vi "EOD Read TEST.vi"(8 "error in (no error)":errorcluster, 11 "Byte Stream File in":refnum<file>) -> (0 "error out":errorcluster, 1 "EODDataOut":T1(array[cluster]), 2 "Iteration Number":i32, 3 "Byte Stream File out":refnum<file>)   [LabVIEW 2014]
panel:
  out "Wave Offset":i32[](array[numeric])
  # "EOD File Reader VI"
  # "Inputs"
  # "Outputs"
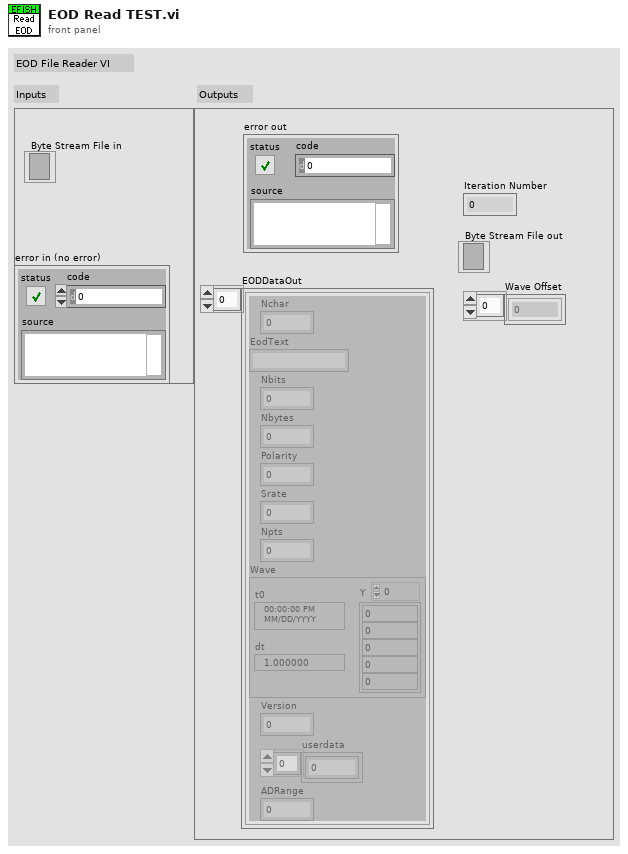
[diagram p1: front panel]
types:
  T1 = cluster{"Nchar":i32, "EodText":string, "Nbits":i32, "Nbytes":i32, "Polarity":i32, "Srate":i32, "Npts":i32, "Wave":waveform(dbl), "Version":i32, "userdata":dbl[], "ADRange":dbl}[]
  T2 = cluster{u8, string, i8, i8, i8, u32, u32, "Waveform":waveform(i16), "Version":i32, sgl[], sgl}
  T3 = cluster{"Nchar":i32, "EodText":string, "Nbits":i32, "Nbytes":i32, "Polarity":i32, "Srate":u32, "Npts":u32, "Wave":waveform(dbl), "Version":i32, "userdata":dbl[], "ADRange":dbl}[]
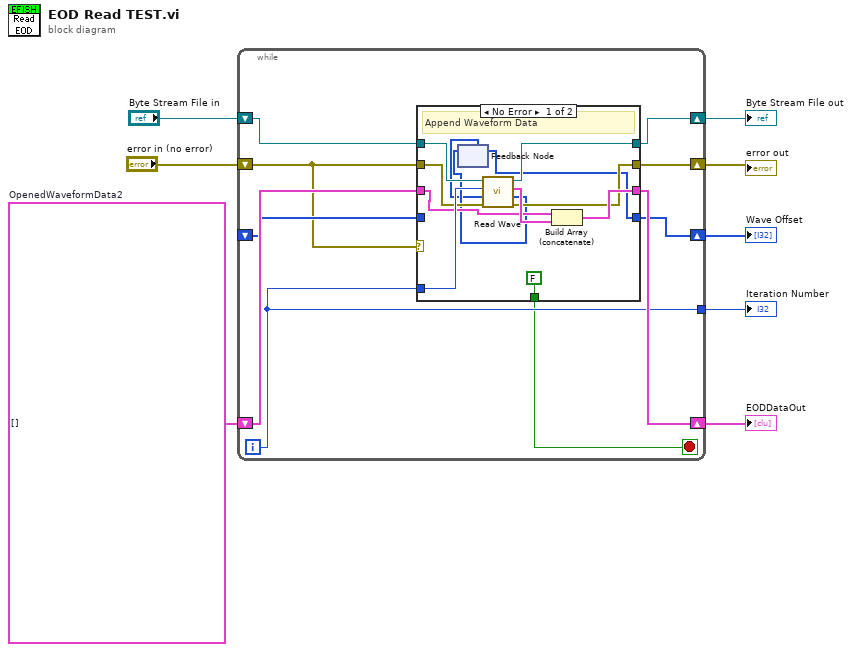
[diagram p0: block diagram]
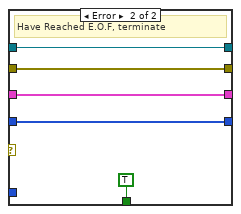
[diagram p2: hidden frame]
diagram:
  w4 = T1 []  # OpenedWaveformData2
  n1 = while {
    shift-right: [w15] -> w6
    shift-left: "Byte Stream File in" -> [w18]
    shift-right: [w14] -> w7
    shift-left: "error in (no error)" -> [w10]
    shift-right: [w16] -> w3
    shift-left: w4 -> [w17]
    shift-right: [w13] -> w2
    shift-left: _ -> [w12]
    tunnel: [w11] -> w1
    i -> [w11]
    stop <- w9 stop-if-true
    n2 = case shown="No Error" w10 {
      tunnel: w11 -> [w29 _]
      tunnel: w10 -> [w28 w32]
      tunnel: w18 -> [w27 w33]
      tunnel: w17 -> [w24 w34]
      tunnel: [w25 w34] -> w16
      tunnel: [w23 w33] -> w15
      tunnel: [w22 w32] -> w14
      tunnel: [w19 w31] -> w13
      tunnel: w12 -> [_ w31]
      tunnel: [FALSE TRUE] -> w9
      frame No Error {
        # "Append Waveform Data"
        n3 = feedback #1() -> (w19:i32[])  [unwired: 1 in]
        n4 = call "Read Wave.vi"("error in"=w28, "Wave Offset Input"=w19, "Iteration of Loop"=w29, "refnum"=w27) -> ("error out"=w22:errorcluster, "Wave Offset"=w20:i32[], "output cluster"=w26:T2, "refnum out"=w23:refnum<file>)  [unwired: 3 in]
        n5 = feedback-in #1(w20) -> ()
        n6 = Build Array (concatenate)(w24, w26) -> (w25:T3)
      }
      frame Error {
        # "Have Reached E.O.F, terminate"
      }
    }
  }
  "error out" <- w7
  "Byte Stream File out" <- w6
  "Iteration Number" <- w1
  "Wave Offset" <- w2
  "EODDataOut" <- w3
